vi "peak finding.vi"() -> ()   [LabVIEW 2019]
uses:
  <vilib>/Utility/file.llb/Read Delimited Spreadsheet (DBL).vi
  <vilib>/measure/mamon.llb/Trigger Detection for 1 Channel.vi
  <vilib>/measure/NI_MAPro.lvlib
panel:
  out "x+1":i32
  out "column count":bool
  out "Numeric 2":i32=1
  out "Numeric":i32=1
  out "error out":errorcluster
  in  "error in":errorcluster
  out "Waveform Graph 2":dbl[][](graph)
  out "subarray":dbl[][](array[numeric])
  out "all rows":dbl[][](array[numeric])
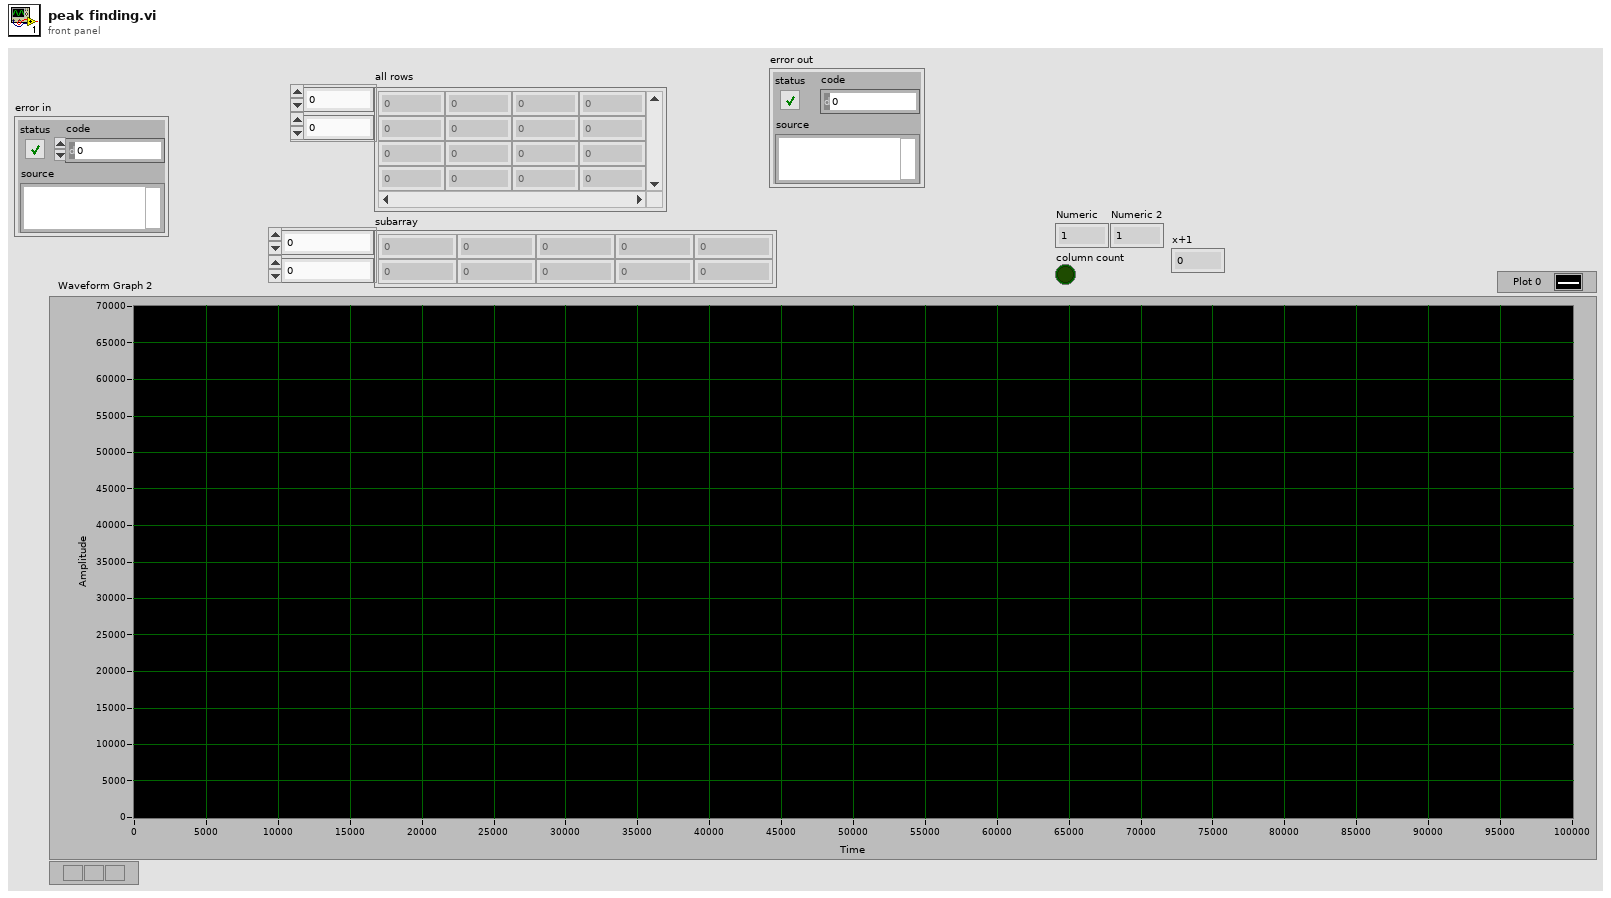
[diagram p1: front panel]
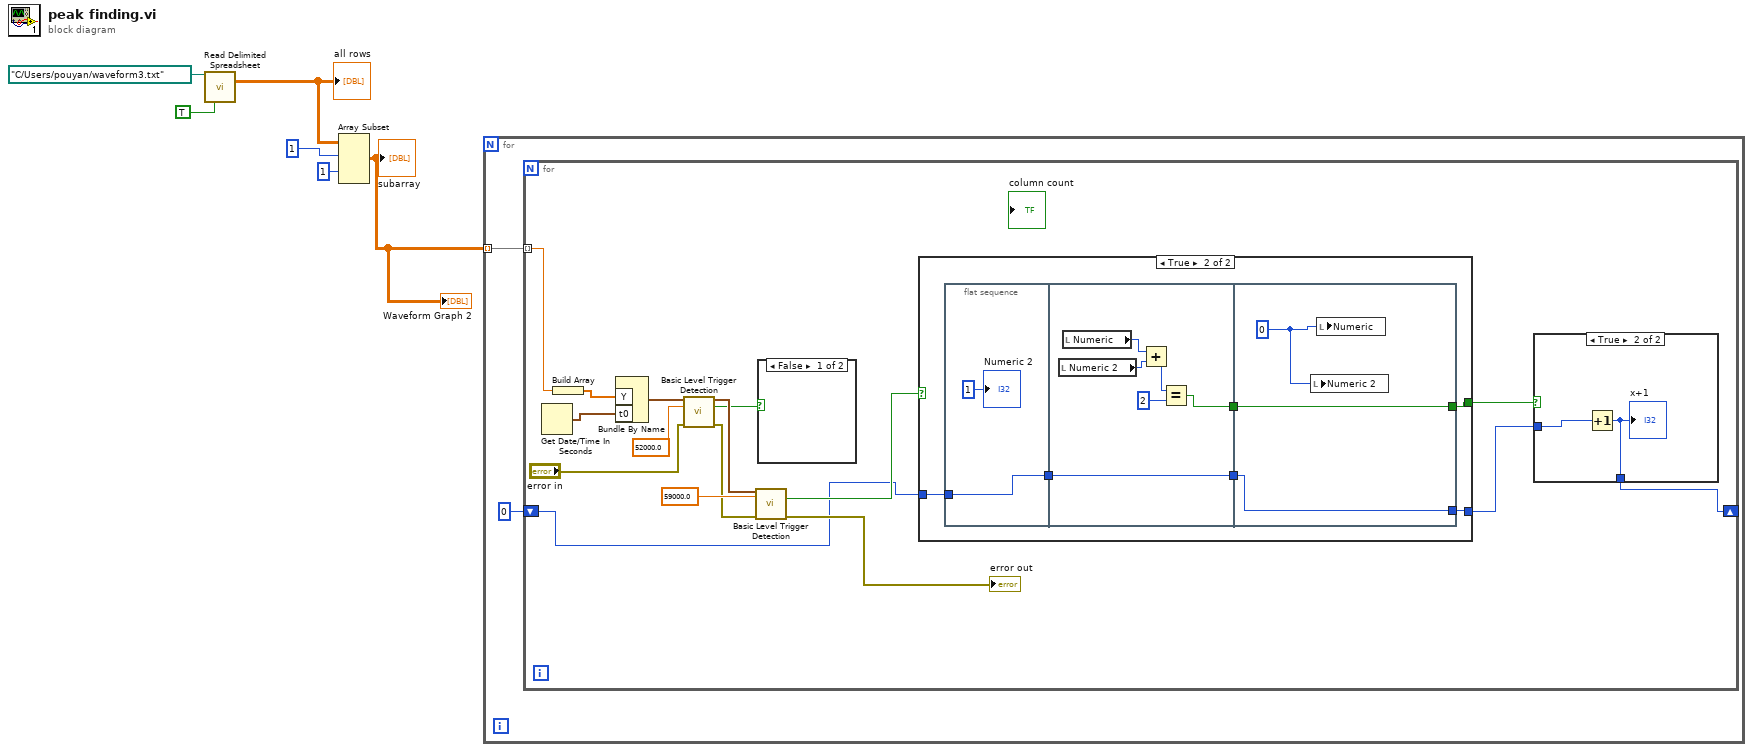
[diagram p0: block diagram]
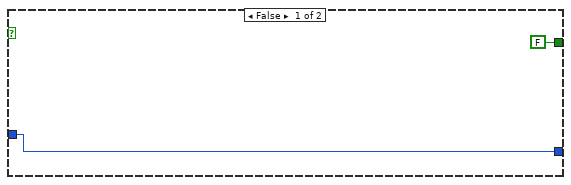
[diagram p3: hidden frame]
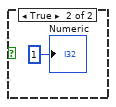
[diagram p4: hidden frame]
diagram:
  n1 = call-poly <vilib>:"Read Delimited Spreadsheet.vi"("file path (dialog if empty)"=path "C:/Users/pouyan/waveform3.txt", "transpose? (F)"=TRUE) -> ("all rows"=w5:dbl[][])  [unwired: 8 in, 5 out]
  "all rows" <- w5
  n2 = Array Subset(array=w5, index (row)=1 ("index"), index (col)=1 ("index")) -> (w2:dbl[][])  [unwired: 2 in]
  "subarray" <- w2
  "Waveform Graph 2" <- w2
  n3 = for {
    tunnel: w2 -> [w8] mode=indexing
    n4 = for {
      tunnel: w8 -> [w15] mode=indexing
      shift-right: [w9] -> _
      shift-left: 0 -> [w12]
      n5 = Get Date/Time In Seconds() -> (seconds since 1Jan1904=w16:timestamp)
      n6 = Build Array(w15) -> (w14:dbl[])
      n7 = Bundle By Name("Y"=w14, "t0"=w16) -> (w21:waveform(dbl))  [unwired: 1 in]
      n8 = call-poly <vilib>:"Basic Level Trigger Detection.vi"("signal in"=w21, "level"=52000.0, "error in (no error)"="error in") -> ("trigger detected?"=w20:bool, "error out"=w19:errorcluster)  [unwired: 10 in, 1 out]
      n9 = call-poly <vilib>:"Basic Level Trigger Detection.vi"("signal in"=w21, "level"=59000.0, "error in (no error)"=w19) -> ("trigger detected?"=w17:bool, "error out"=→"error out":errorcluster)  [unwired: 10 in, 1 out]
      n10 = case shown="False" w20 {
        frame False {
        }
        frame True {
          "Numeric" <- 1
        }
      }
      n11 = case shown="True" w17 {
        tunnel: w12 -> [w28 w31]
        tunnel: [w28 w30] -> w10
        tunnel: [FALSE w29] -> w11
        frame False {
        }
        frame True {
          n12 = flat-sequence {
            tunnel: [w35] -> w32
            tunnel: w31 -> [w35]
            tunnel: [w38] -> w34
            tunnel: [w37] -> w33
            tunnel: w32 -> [w37]
            tunnel: [w45] -> w29
            tunnel: w34 -> [w45]
            tunnel: w33 -> [w43]
            tunnel: [w43] -> w30
            frame #0 {
              "Numeric 2" <- 1
            }
            frame #1 {
              n13 = local read "Numeric 2"() -> (w41:i32)
              n14 = local read "Numeric"() -> (w42:i32)
              n15 = Add(x=w42, y=w41) -> (x+y=w40:i32)
              n16 = Equal?(x=w40, y=2) -> (x = y?=w38:bool)
            }
            frame #2 {
              w44 = 0 ("Numeric")
              n17 = local write "Numeric 2"(w44) -> ()
              n18 = local write "Numeric"(w44) -> ()
            }
          }
        }
      }
      n19 = case shown="True" w11 {
        tunnel: w10 -> [w24 w26]
        tunnel: [w24 w25] -> w9
        frame False {
        }
        frame True {
          n20 = Increment(x=w26) -> (x+1=w25:i32)
          "x+1" <- w25
        }
      }
    }
  }
